vi "dynamicstackplots.vi"() -> ()   [LabVIEW 2013]
doc: "This VI dynamically stacks plots on the front panel. The front panel contains an array of clusters, and each cluster contains a waveform chart. The VI bundles the generated data array into a cluster for each dynamic plot. The VI then groups all clusters together into an array and passes them to the array on the front panel. The VI also makes sure all dynamic plots are visible on the front panel."
uses:
  <vilib>/Analysis/NI_AALBase.lvlib
panel:
  out "Array":cluster{"Waveform Chart":dbl[]}[](array[cluster]) caption="Array of clusters, each containing one waveform chart"
  in  "Number of Stacked Plots":i32
  in  "Stop":bool
  # "Select Help»Show Context Help and move the cursor over the VI icon to display help for this VI."
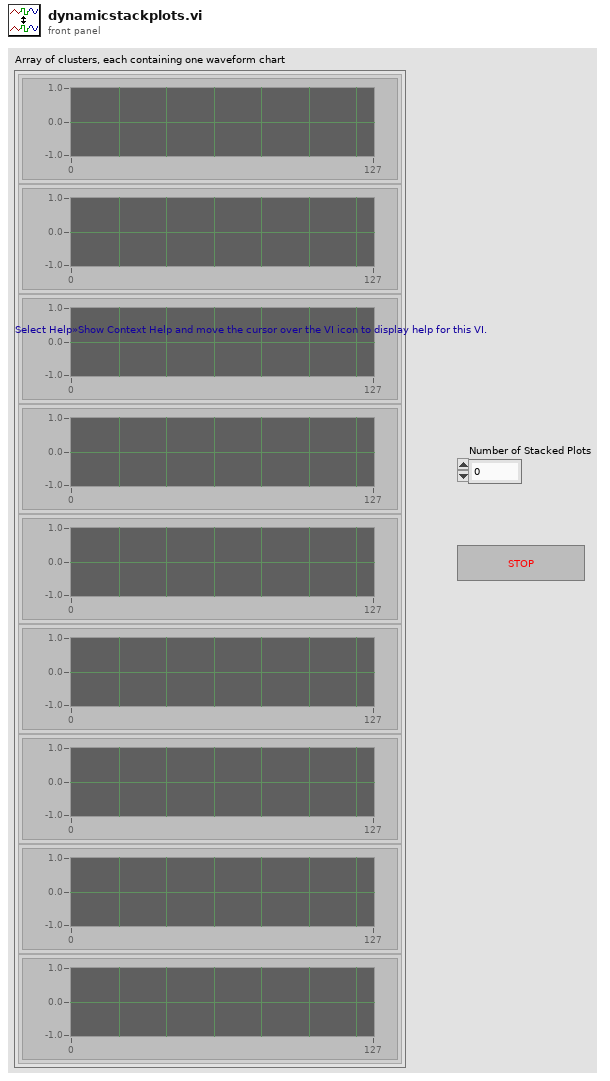
[diagram p1: front panel]
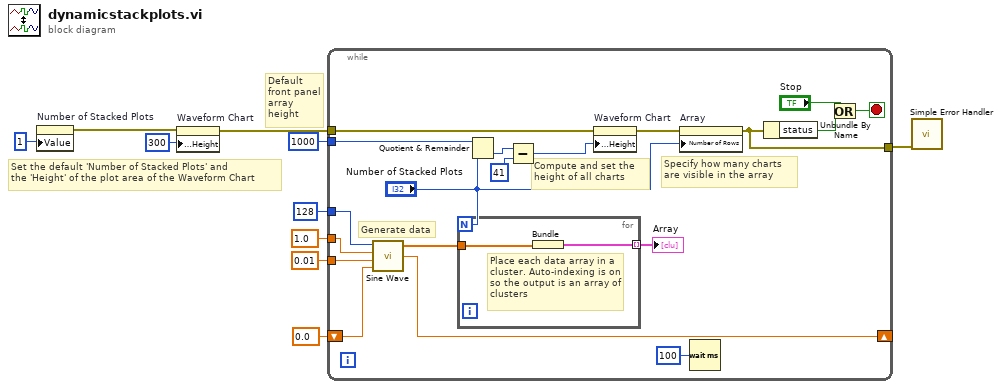
[diagram p0: block diagram]
diagram:
  # "Default front panel array height"
  # "Set the default 'Number of Stacked Plots' and\nthe 'Height' of the plot area of the Waveform Chart"
  n1 = property on="Number of Stacked Plots" class="DigNum (strict)"("Value"=1 ("Number of Stacked Plots")) -> (error out=w4:errorcluster)  [unwired: 2 in, 1 out]
  n2 = property on="Waveform Chart" class="WFGraph (strict)"(error in=w4, "Plot Area:Size:Height"=u32 300) -> (error out=w3:errorcluster)  [unwired: 1 in, 1 out]
  n3 = while {
    tunnel: w3 -> [w17]
    tunnel: u32 1000 ("Height") -> [w21]
    tunnel: 0.01 ("f") -> [w23]
    tunnel: 1.0 ("amplitude") -> [w24]
    tunnel: 128 ("samples") -> [w25]
    shift-left: 0.0 -> [w28]
    shift-right: [w22] -> _
    tunnel: [w11] -> w1
    stop <- w12 stop-if-true
    # "Generate data"
    # "Specify how many charts\nare visible in the array"
    # "Compute and set the \nheight of all charts"
    n4 = call <vilib>:"Sine Wave.vi"("samples"=w25, "amplitude"=w24, "frequency"=w23, "phase in"=w28) -> ("sine wave"=w27:dbl[], "phase out"=w22:dbl)  [unwired: 1 in, 1 out]
    n5 = for {
      N: "Number of Stacked Plots" -> [_]
      tunnel: [w31] -> w26 mode=indexing
      tunnel: w27 -> [w30]
      # "Place each data array in a cluster. Auto-indexing is on so the output is an array of clusters"
      n6 = Bundle("sine wave"=w30) -> (w31:cluster{"sine wave":dbl[]})  [unwired: 1 in]
    }
    "Array" <- w26
    n7 = Quotient & Remainder(x=w21, y="Number of Stacked Plots") -> (floor(x/y)=w20:u32)  [unwired: 1 out]
    n8 = Subtract(x=w20, y=u32 41) -> (x-y=w16:u32)
    n9 = property on="Waveform Chart" class="WFGraph (strict)"(error in=w17, "Plot Area:Size:Height"=w16) -> (error out=w18:errorcluster)  [unwired: 1 in, 1 out]
    n10 = property on="Array" class="Arr (strict)"(error in=w18, "Number of Rows"="Number of Stacked Plots") -> (error out=w11:errorcluster)  [unwired: 1 in, 1 out]
    n11 = Wait (ms)(milliseconds to wait=u32 100) -> ()  [unwired: 1 out]
    n12 = Unbundle By Name(w11) -> ("status"=w13:bool)
    n13 = Or(x="Stop", y=w13) -> (x .or. y?=w12:bool)
  }
  n14 = call <vilib>:"Simple Error Handler.vi"("error in (no error)"=w1) -> ()  [unwired: 4 in, 5 out]
